vi "ReadText.vi"(8 "Error In":errorcluster) -> (0 "Error Out":errorcluster, 2 "TextOut":string)   [LabVIEW 2020, in "Console.lvclass"]
uses:
  Console.lvclass
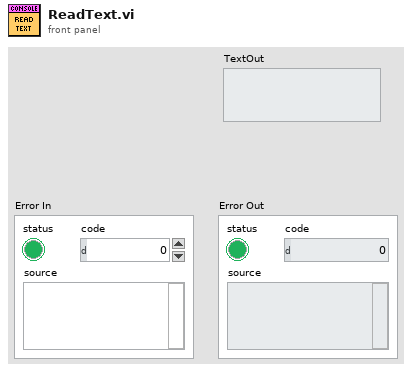
[diagram p1: front panel]
types:
  T1 = typedef "Console.lvclass/ObjectAttributes.ctl" = cluster{"ConsoleText":string[]}
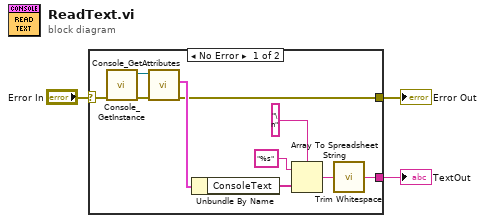
[diagram p0: block diagram]
diagram:
  n1 = case shown="No Error" "Error In" {
    selector: "Error In" -> [w10 w14]
    tunnel: [w12 w14] -> w2
    tunnel: [w4 _] -> w1
    frame No Error {
      n2 = call "Console_GetInstance.vi"("error in"=w10) -> ("error out"=w9:errorcluster, "reference out"=w11:refnum<class "Console.lvclass">)  [unwired: 6 in, 3 out]
      n3 = call "Console_GetAttributes.vi"("error in (no error)"=w9, "reference in"=w11) -> ("error out"=w12:errorcluster, "Data"=w13:T1)  [unwired: 6 in, 2 out]
      n4 = Unbundle By Name(w13) -> ("ConsoleText"=w6:string[])
      n5 = Array To Spreadsheet String(delimiter (Tab)="\n", array=w6, 3:"%s" ("format string")) -> (spreadsheet string=w5:string)
      n6 = call <vilib>:"Trim Whitespace.vi"("string"=w5) -> ("trimmed string"=w4:string)  [unwired: 1 in]
    }
    frame Error {
    }
  }
  "Error Out" <- w2
  "TextOut" <- w1
